vi "201_radar_objs.vi"(11 "201":string) -> (3 "radar_objs":cdb[](array[numeric]))   [LabVIEW 2022 SP3]
panel:
  out "[]Array":string[](array[string])
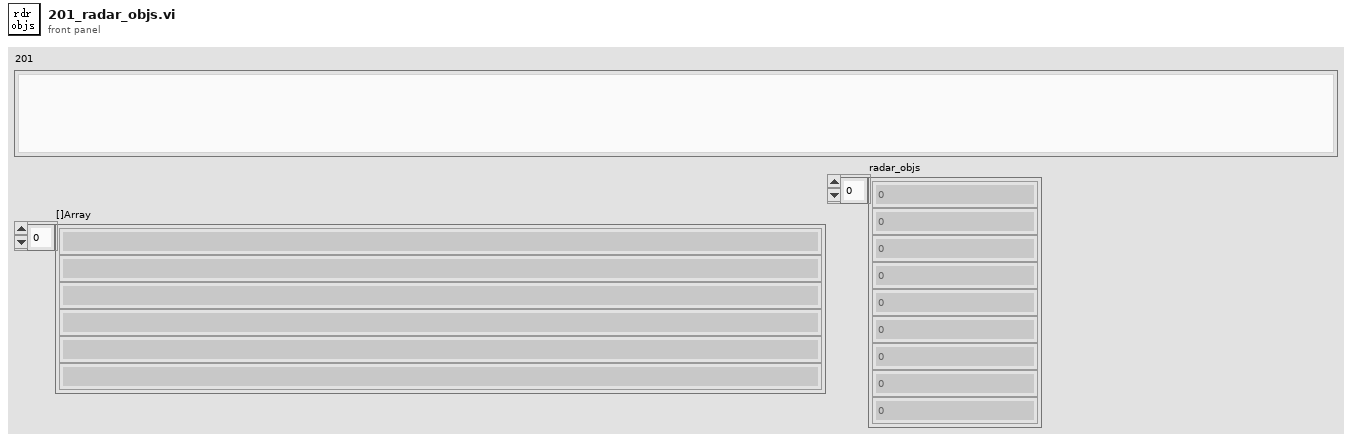
[diagram p1: front panel]
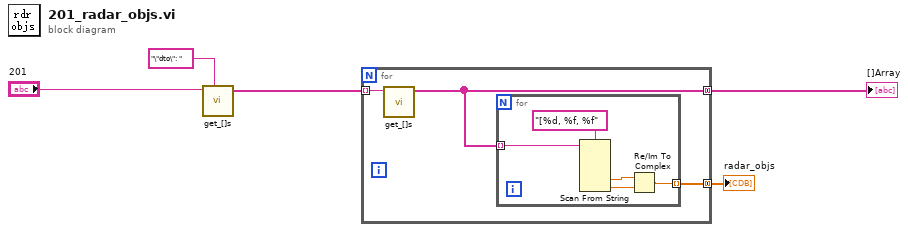
[diagram p0: block diagram]
diagram:
  n1 = call "get_[]s.vi"("prefix"="\"dto\": ", "String"="201") -> ("[]Array"=w3:string[])  [unwired: 9 in]
  n2 = for {
    tunnel: w3 -> [w8] mode=indexing
    tunnel: [w7] -> w5 mode=concatenating
    tunnel: [w6] -> w1 mode=concatenating
    n3 = call "get_[]s.vi"("String"=w8) -> ("[]Array"=w7:string[])  [unwired: 10 in]
    n4 = for {
      tunnel: w7 -> [w13] mode=indexing
      tunnel: [w9] -> w6 mode=indexing
      n5 = Scan From String(format string="[%d, %f, %f", input string=w13) -> (output 2=w10:dbl, output 3=w11:dbl)  [unwired: 6 in, 3 out]
      n6 = Re/Im To Complex(1:w11, 2:w10) -> (0:w9:cdb)
    }
  }
  "[]Array" <- w5
  "radar_objs" <- w1
